vi "Average_while_loop.vi"() -> ()   [LabVIEW 2015]
panel:
  in  "stop":bool
  out "Waveform Chart":cluster{"number: 0 to 1":dbl, dbl}(graph)
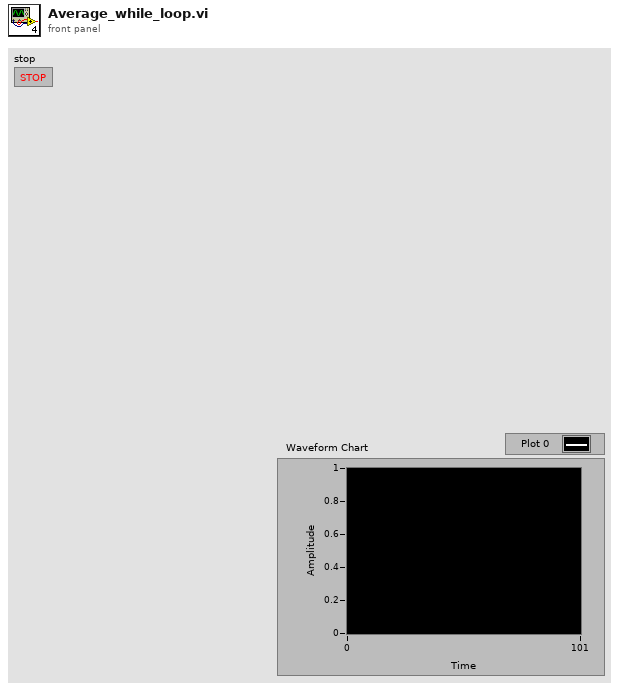
[diagram p1: front panel]
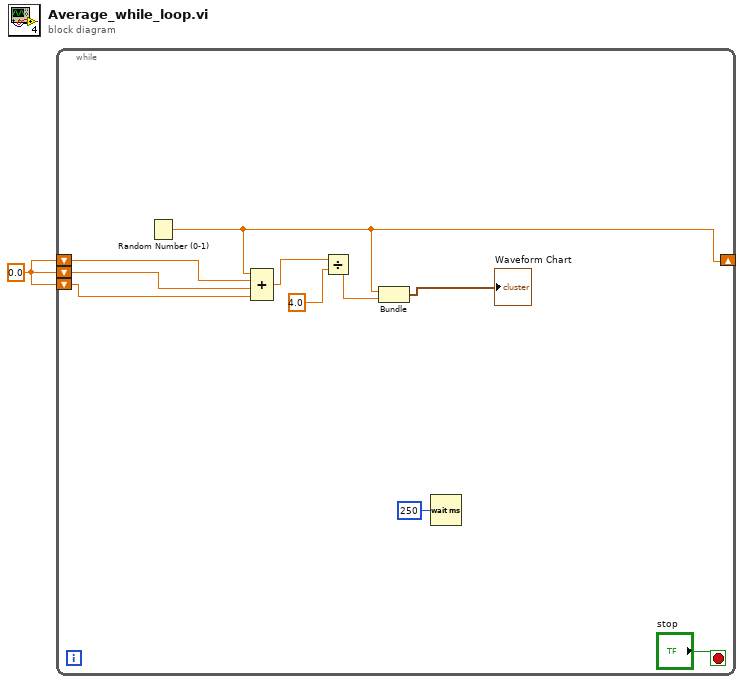
[diagram p0: block diagram]
diagram:
  w1 = 0.0 ("number: 0 to 1")
  n1 = while {
    shift-right: [w6] -> _
    shift-left: w1 -> [w9]
    shift-left: w1 -> [w8]
    shift-left: w1 -> [w7]
    stop <- "stop" stop-if-true
    n2 = Random Number (0-1)() -> (number: 0 to 1=w6:dbl)
    n3 = Compound Arithmetic op=ADD(w6, w9, w8, w7) -> (w11:dbl)
    n4 = Divide(x=w11, y=4.0) -> (x/y=w5:dbl)
    n5 = Bundle("number: 0 to 1"=w6, w5) -> (→"Waveform Chart":cluster{"number: 0 to 1":dbl, dbl})  [unwired: 1 in]
    n6 = Wait (ms)(milliseconds to wait=u32 250) -> ()  [unwired: 1 out]
  }
